vi "Generate Standard VI HTML Documentation.vi"(4 "Root Folder Name":string="Toolkit", 5 "Images Destination":path=path "", 6 "Requirement":string="Labstache", 7 "Destination":path=path "", 8 "Error In":errorcluster, 11 "VI":path=path "") -> (0 "Error Out":errorcluster)   [LabVIEW 2018, in "Scripts.lvlib"]
uses:
  Scripts.lvlib
  Toolkit/Data/Array/Array.lvclass
  D:/Users/cfield/Code/Field R&D Services/Mustache/LabVIEW/trunk/src/Toolkit/Data/Datum/Datum.lvclass
  Toolkit/Data/Map/Map.lvclass
  Toolkit/Data/Map/Support/From String.vi
  Toolkit/Data/Map/Support/From Datum.vi
  Toolkit/Data/Map/Support/From Map Array.vi
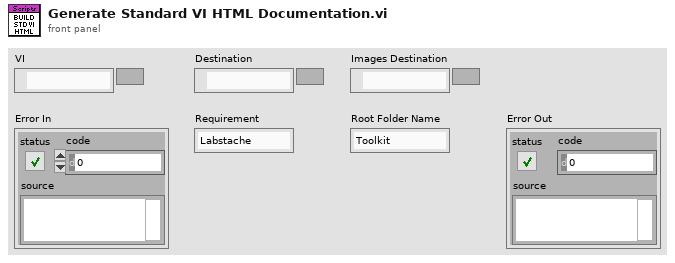
[diagram p1: front panel]
types:
  T1 = cluster{"Alt":string, "Description":string, "Src":string}[]
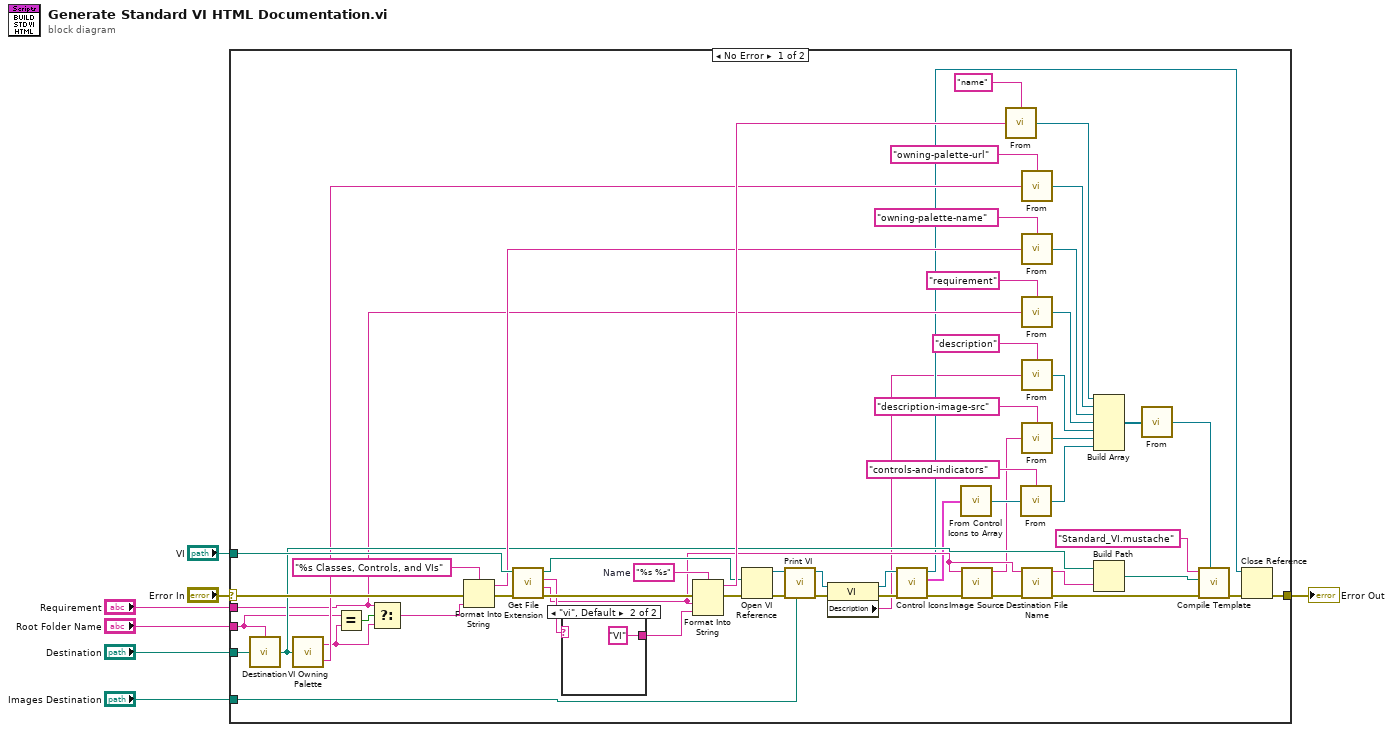
[diagram p0: block diagram]
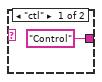
[diagram p2: hidden frame]
diagram:
  n1 = case shown="No Error" "Error In" {
    selector: "Error In" -> [w53 w67]
    tunnel: [w43 w67] -> w7
    tunnel: "VI" -> [w58 _]
    tunnel: "Destination" -> [w57 _]
    tunnel: "Requirement" -> [w49 _]
    tunnel: "Images Destination" -> [w45 _]
    tunnel: "Root Folder Name" -> [w8 _]
    frame No Error {
      w61 = "%s %s"  # Name
      n2 = call "Destination.vi"("Root Destination In"=w57, "Root Folder Name"=w8) -> ("Root Destination Out"=w52:path)
      n3 = call "VI Owning Palette.vi"("Destination"=w52) -> ("Name"=w48:string, "URL"=w51:string)
      n4 = Equal?(x=w8, y=w48) -> (x = y?=w50:bool)
      n5 = Select(t=w49, s=w50, f=w48) -> (s? t:f=w47:string)
      n6 = Format Into String(format string="%s Classes, Controls, and VIs", error in=w53, w47) -> (resulting string=w54:string, error out=w56:errorcluster)  [unwired: 1 in]
      n7 = call <vilib>:"Get File Extension.vi"("error in (no error)"=w56, "file"=w58) -> ("error out"=w62:errorcluster, "filename without extension"=w46:string, "lowercase file extension"=w60:string, "dup file"=w59:path)  [unwired: 5 in, 1 out]
      n8 = case shown="\"vi\", Default" w60 {
        tunnel: ["Control" "VI"] -> w63
        frame "ctl" {
        }
        frame "vi", Default {
        }
      }
      n9 = Format Into String(format string=w61, error in=w62, w46, w63) -> (resulting string=w64:string, error out=w44:errorcluster)  [unwired: 1 in]
      n10 = Open VI Reference(vi path=w59, error in (no error)=w44) -> (vi reference=w42:refnum<vi>, error out=w39:errorcluster)  [unwired: 4 in]
      n11 = call "Print VI.vi"("Images Destination"=w45, "Error In"=w39, "VI In"=w42) -> ("Error Out"=w40:errorcluster, "VI Out"=w41:refnum<vi>)  [unwired: 7 in]
      n12 = property class="VI"(reference=w41, error in=w40) -> (reference out=w36:refnum<vi>, error out=w29:errorcluster, "Description"=w18:string)
      n13 = call "Control Icons.vi"("Error In"=w29, "VI In"=w36) -> ("Error Out"=w10:errorcluster, "Control Icons"=w15:T1, "VI Out"=w38:refnum<vi>)  [unwired: 7 in]
      n14 = call "From Control Icons to Array.vi"("Control Icons"=w15) -> ("Array"=w35:refnum<class "Array.lvclass">)
      n15 = call "Image Source.vi"("Error In"=w10, "Spaced File Stem"=w46) -> ("Error Out"=w11:errorcluster, "Image Src"=w20:string)  [unwired: 8 in]
      n16 = call-poly "From.vi"("Value"=w64, "Key"="name") -> ("Map"=w28:refnum<class "Map.lvclass">)
      n17 = call-poly "From.vi"("Value"=w35, "Key"="controls-and-indicators") -> ("Map"=w25:refnum<class "Map.lvclass">)
      n18 = call-poly "From.vi"("Value"=w51, "Key"="owning-palette-url") -> ("Map"=w34:refnum<class "Map.lvclass">)
      n19 = call-poly "From.vi"("Value"=w54, "Key"="owning-palette-name") -> ("Map"=w32:refnum<class "Map.lvclass">)
      n20 = call-poly "From.vi"("Value"=w49, "Key"="requirement") -> ("Map"=w30:refnum<class "Map.lvclass">)
      n21 = call-poly "From.vi"("Value"=w18, "Key"="description") -> ("Map"=w27:refnum<class "Map.lvclass">)
      n22 = call-poly "From.vi"("Value"=w20, "Key"="description-image-src") -> ("Map"=w26:refnum<class "Map.lvclass">)
      n23 = call "Destination File Name.vi"("Error In"=w11, "File Stem"=w46) -> ("Error Out"=w24:errorcluster, "Destination File Name"=w16:string)  [unwired: 8 in]
      n24 = Build Array(w28, w34, w32, w30, w27, w26, w25) -> (w14:refnum<class "Map.lvclass">[])
      n25 = Build Path(base path=w52, name or relative path=w16) -> (appended path=w12:path)
      n26 = call-poly "From.vi"("Maps"=w14) -> ("Map"=w13:refnum<class "Map.lvclass">)  [unwired: 1 in]
      n27 = call "Compile Template.vi"("Data"=w13, "Error In"=w24, "Output"=w12, "Template File Name"="Standard_VI.mustache" ("name or relative path")) -> ("Error Out"=w37:errorcluster)  [unwired: 7 in]
      n28 = Close Reference(reference=w38, error in (no error)=w37) -> (error out=w43:errorcluster)
    }
    frame Error {
    }
  }
  "Error Out" <- w7
